vi "GetPipleLineImageBuffer.vi"(8 "error in (no error)":errorcluster, 11 "Microscope in":refnum<class "Microscope.lvclass">) -> (0 "error out":errorcluster, 2 "PiplelineImageBuffers":refnum<queue>, 3 "Microscope out":refnum<class "Microscope.lvclass">)   [LabVIEW 2020, in "Microscope.lvlib" / "Microscope.lvclass"]
uses:
  Microscope.lvclass
  <vilib>/vision/Image Controls.llb/IMAQ Image.ctl
  Microscope.lvclass/Microscope.ctl
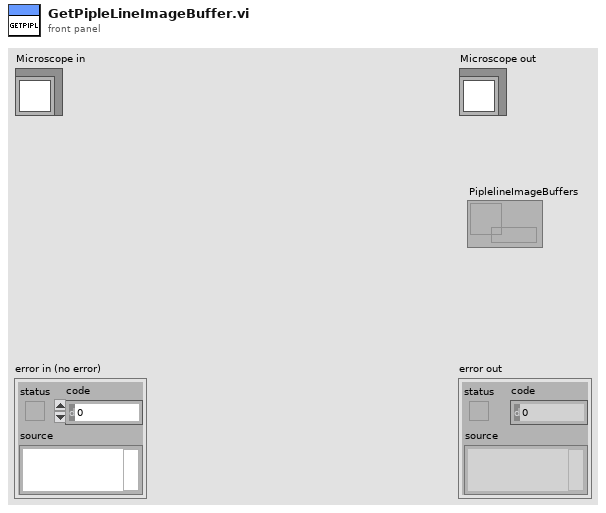
[diagram p1: front panel]
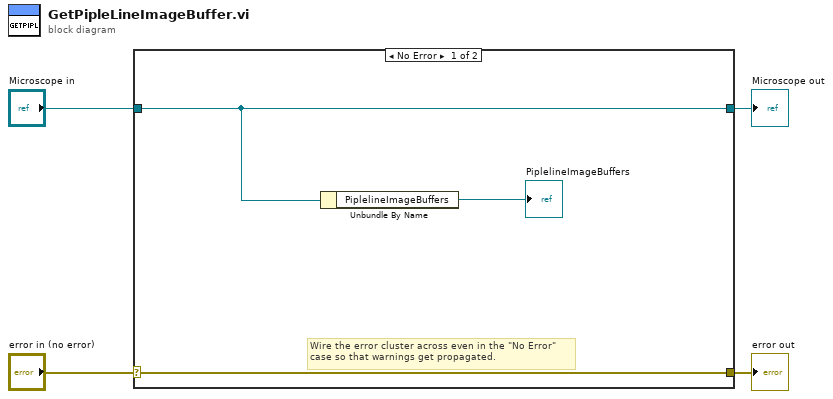
[diagram p0: block diagram]
diagram:
  n1 = case shown="No Error" "error in (no error)" {
    selector: "error in (no error)" -> [w7 w9]
    tunnel: [w7 w9] -> w3
    tunnel: [w6 w8] -> w1
    tunnel: "Microscope in" -> [w6 w8]
    frame No Error {
      # "Wire the error cluster across even in the \"No Error\"\ncase so that warnings get propagated."
      n2 = Unbundle By Name(w6) -> ("PiplelineImageBuffers"=→"PiplelineImageBuffers":refnum<queue>)
    }
    frame Error {
    }
  }
  "error out" <- w3
  "Microscope out" <- w1
